vi "aal_moving average with decimation by order (complex input).vi"(1 "Reset":bool, 2 "N":i32=1, 3 "x":cdb[](array[numeric])) -> (0 "y":cdb[](array[numeric]))   [LabVIEW 2018, in "NI_AALPro.lvlib"]
uses:
  <vilib>/Analysis/NI_AALPro.lvlib
  <resource>/lvanlys.dll
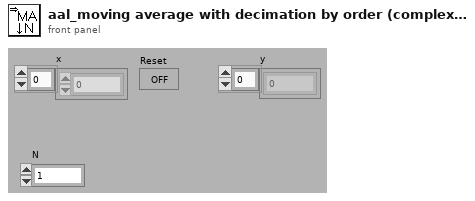
[diagram p1: front panel]
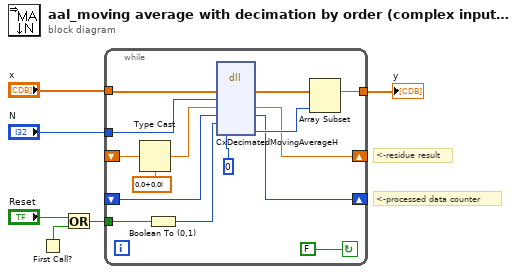
[diagram p0: block diagram]
diagram:
  # "<-processed data counter"
  # "<-residue result"
  n1 = First Call?() -> (First Call?: T/F=w3:bool)
  n2 = Or(x="Reset", y=w3) -> (x .or. y?=w5:bool)
  n3 = while {
    tunnel: [w18] -> w1
    tunnel: "N" -> [w16]
    tunnel: w5 -> [w21]
    tunnel: "x" -> [w20]
    shift-left: _ -> [w11]
    shift-right: [w9] -> _
    shift-left: _ -> [w15]
    shift-right: [w10] -> _
    stop <- FALSE continue-if-true
    n4 = Type Cast(type=cdb 0.0+0.0i, x=w15) -> (*(type *) &x=w8:cdb)
    n5 = Boolean To (0,1)(Boolean=w21) -> (0, 1=w14:i16)
    n6 = dll-call lib="C:/Program Files (x86)/National Instruments/LabVIEW 2018/resource/lvanlys.*" fn="CxDecimatedMovingAverageH"("x"=w20, "N"=w16, w8, "cnt"=w11, "reset"=w14, "out_len"=0 ("yH")) -> ("x"=w19:cdb[], w10:cdb, "cnt"=w9:i32, "out_len"=w12:i32)  [unwired: 6 in, 2 out]
    n7 = Array Subset(array=w19, length=w12) -> (w18:cdb[])  [unwired: 1 in]
  }
  "y" <- w1
